vi "Run Test.vi"(8 "error in (no error)":errorcluster, 10 "Measurement Name":string, 11 "Test Framework in":refnum<class "Test Framework.lvclass">) -> (0 "error out":errorcluster, 2 "Canceled":bool, 3 "Test Framework out":refnum<class "Test Framework.lvclass">)   [LabVIEW 2020, in "Test Framework.lvclass"]
uses:
  Test Framework.lvclass
  Instruments/Instrument.lvclass
  Test Framework.lvclass/Test Framework.ctl
  Measurements/Measurement.lvclass/Measurement.ctl
  Instruments/Temperature Control/Temperature Control.lvclass
  C:/Sandbox/RF Bench/Source Code/WiSpry Test Framework/Instruments/Instrument.lvclass
  Instruments/Power Supply/Power Supply.lvclass
  Measurements/Measurement.lvclass
  XML Handler/XML Handler.lvclass
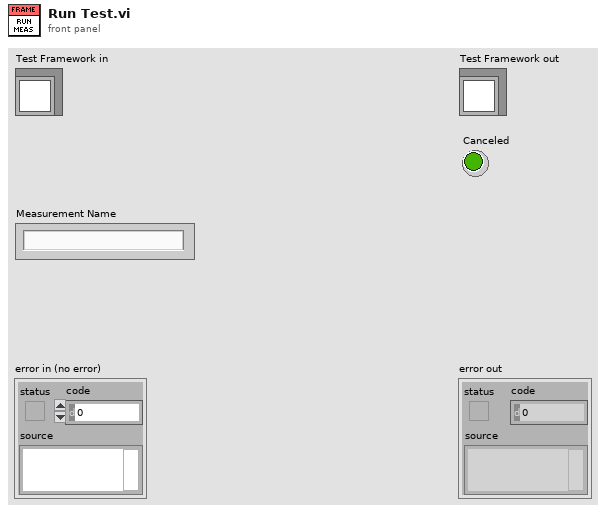
[diagram p1: front panel]
types:
  T1 = cluster{"Instrument Name":string, "Instrument.lvclass":refnum<class "Instrument.lvclass">, "Reference":bool}[]
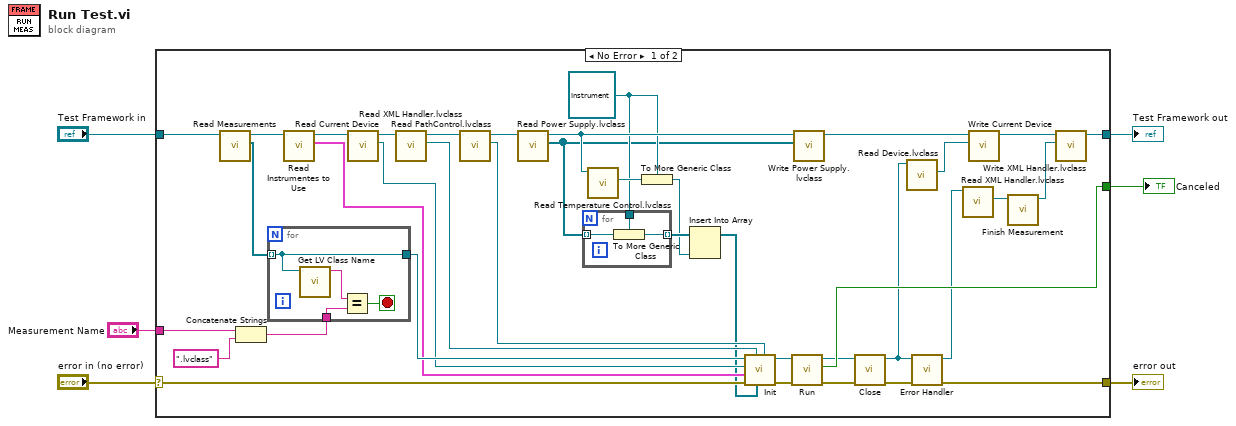
[diagram p0: block diagram]
diagram:
  n1 = case shown="No Error" "error in (no error)" {
    selector: "error in (no error)" -> [w36 w53]
    tunnel: [w15 w53] -> w5
    tunnel: [w24 w52] -> w3
    tunnel: "Test Framework in" -> [w44 w52]
    tunnel: "Measurement Name" -> [w42 _]
    tunnel: [w35 _] -> w1
    frame No Error {
      w18 = refnum<class "Instrument.lvclass"> refnum ("Instrument.lvclass")
      n2 = call "Read Measurements.vi"("Test Framework in"=w44) -> ("Measurements"=w43:refnum<class "Measurement.lvclass">[], "Test Framework out"=w34:refnum<class "Test Framework.lvclass">)  [unwired: 9 in]
      n3 = Concatenate Strings(w42, ".lvclass" ("string")) -> (w40:string)
      n4 = for {
        tunnel: w43 -> [w48] mode=indexing
        tunnel: w40 -> [w50]
        tunnel: [w48] -> w39
        stop <- w49 stop-if-true
        n5 = call <vilib>:"Get LV Class Name.vi"("object"=w48) -> ("class name"=w51:string)  [unwired: 9 in, 1 out]
        n6 = Equal?(x=w51, y=w50) -> (x = y?=w49:bool)
      }
      n7 = call "Read Instrumentes to Use.vi"("Test Framework in"=w34) -> ("Instrumentes to Use"=w33:T1, "Test Framework out"=w32:refnum<class "Test Framework.lvclass">)  [unwired: 9 in]
      n8 = call-dynamic "Read Current Device.vi"("Test Framework in"=w32) -> ("Current Device.lvclass"=w31:refnum<class "Device.lvclass">, "Test Framework out"=w30:refnum<class "Test Framework.lvclass">)  [unwired: 9 in]
      n9 = call "Read XML Handler.lvclass.vi"("Test Framework in"=w30) -> ("XML Handler.lvclass"=w29:refnum<class "XML Handler.lvclass">, "Test Framework out"=w28:refnum<class "Test Framework.lvclass">)  [unwired: 9 in]
      n10 = call "Read PathControl.lvclass.vi"("Test Framework in"=w28) -> ("PathControl.lvclass"=w27:refnum<class "PathControl.lvclass">, "Test Framework out"=w22:refnum<class "Test Framework.lvclass">)  [unwired: 9 in]
      n11 = call "Read Power Supply.lvclass.vi"("Test Framework in"=w22) -> ("Power Supply lvclasses"=w14:refnum<class "Power Supply.lvclass">[], "Test Framework out"=w21:refnum<class "Test Framework.lvclass">)  [unwired: 9 in]
      n12 = for {
        tunnel: w14 -> [w47] mode=indexing
        tunnel: w18 -> [w46]
        tunnel: [w45] -> w20 mode=indexing
        n13 = To More Generic Class(target class=w46, reference=w47) -> (generic class reference=w45:refnum<class "Instrument.lvclass">)
      }
      n14 = call "Read Temperature Control.lvclass.vi"("Test Framework in"=w21) -> ("Temperature Control.lvclass"=w19:refnum<class "Temperature Control.lvclass">)  [unwired: 9 in, 1 out]
      n15 = To More Generic Class(target class=w18, reference=w19) -> (generic class reference=w17:refnum<class "Instrument.lvclass">)
      n16 = Insert Into Array(array=w20, new element=w17) -> (w16:refnum<class "Instrument.lvclass">[])  [unwired: 1 in]
      n17 = call-dynamic "Init.vi"("PathControl.lvclass"=w27, "Environmental classes"=w16, "XML Handler.lvclass"=w29, "error in (no error)"=w36, "Instruments to Use"=w33, "Device.lvclass"=w31, "Measurements in"=w39) -> ("error out"=w37:errorcluster, "Measurements out"=w38:refnum<class "Measurement.lvclass">)  [unwired: 3 in]
      n18 = call-dynamic "Run.vi"("error in (no error)"=w37, "Measurements in"=w38) -> ("error out"=w13:errorcluster, "Canceled"=w35:bool, "Measurements out"=w12:refnum<class "Measurement.lvclass">)  [unwired: 6 in, 1 out]
      n19 = call "Write Power Supply.lvclass.vi"("Power Supply lvclasses"=w14, "Test Framework in"=w21) -> ("Test Framework out"=w8:refnum<class "Test Framework.lvclass">)  [unwired: 9 in]
      n20 = call-dynamic "Close.vi"("error in (no error)"=w13, "Measurements in"=w12) -> ("error out"=w11:errorcluster, "Measurements out"=w10:refnum<class "Measurement.lvclass">)  [unwired: 8 in]
      n21 = call "Read Device.lvclass.vi"("Measurements in"=w10) -> ("Device.lvclass"=w9:refnum<class "Device.lvclass">)  [unwired: 9 in, 1 out]
      n22 = call-dynamic "Error Handler.vi"("error in (no error)"=w11, "Measurements in"=w10) -> ("error out"=w15:errorcluster, "Measurements out"=w26:refnum<class "Measurement.lvclass">)  [unwired: 7 in, 1 out]
      n23 = call "Read XML Handler.lvclass.vi"("Measurements in"=w26) -> ("XML Handler.lvclass"=w25:refnum<class "XML Handler.lvclass">)  [unwired: 9 in, 1 out]
      n24 = call-dynamic "Write Current Device.vi"("Current Device.lvclass"=w9, "Test Framework in"=w8) -> ("Test Framework out"=w7:refnum<class "Test Framework.lvclass">)  [unwired: 9 in]
      n25 = call-dynamic "Finish Measurement.vi"("XML Handler in"=w25) -> ("XML Handler out"=w23:refnum<class "XML Handler.lvclass">)  [unwired: 9 in, 1 out]
      n26 = call "Write XML Handler.lvclass.vi"("XML Handler.lvclass"=w23, "Test Framework in"=w7) -> ("Test Framework out"=w24:refnum<class "Test Framework.lvclass">)  [unwired: 9 in]
    }
    frame Error {
    }
  }
  "error out" <- w5
  "Test Framework out" <- w3
  "Canceled" <- w1
